vi "Platform.vi"() -> ()   [LabVIEW 2013]
uses:
  <vilib>/userdefined/High Color/IMAQdx.ctl
  <vilib>/Instr/_visa.llb/VISA Configure Serial Port (Instr).vi
  <vilib>/vision/driver/NI_Vision_Acquisition_Software.lvlib
  <vilib>/vision/NI_Vision_Development_Module.lvlib
panel:
  in  "VISA resource name 3":refnum<visa-resource-name>="COM13" caption="蓝牙串口选择"
  in  "baud rate  3":u16(ring)=9600 caption="蓝牙波特率设置" items=["115200"=0, "57600"=57600, "38400"=38400, "19200"=19200, "9600"=9600]
  out "x = y? 6":bool
  out "x = y? 5":bool
  out "x = y? 4":bool
  out "x = y? 3":bool
  out "x = y? 2":bool
  out "x = y?":bool
  out "数字":i32
  out "当前系统时间":string
  in  "系统总开关":bool
  out "x":i32 min=0 max=1 step=1
  out "检测目标总数目":dbl(knob) scale=0.0..10.0
  in  "连接确认":bool
  out "发送的坐标数据":string
  in  "过滤识别选项":u16(ring)=1 items=["过滤并分类摆放"=4, "过滤矩形目标"=3, "过滤圆形目标"=2, "全部识别"=1]
  in  "baud rate":u16(ring)=9600 caption="通讯波特率设置" items=["115200"=0, "57600"=57600, "38400"=38400, "19200"=19200, "9600"=9600]
  in  "VISA resource name":refnum<visa-resource-name>="COM3" caption="串口号选择"
  out "串口接收区：":string
  out "中间量":string
  in  "清空接收区":bool
  in  "关闭串口（调试）":bool
  in  "空载速率":dbl=1.0 min=1.0 max=3.0 step=1.0
  in  "运行速率":dbl=1.0 min=1.0 max=3.0 step=1.0
  in  "采集相机选择":T1="cam1"
  in  "环境光阈值设置":cluster{"环境光阈值设置":sgl, "上限值 value":sgl}={"环境光阈值设置"=137.0, "上限值 value"=255.0} {"环境光阈值设置" min=0 max=255 step=1 scale=0.0..255.0}
  out "图像处理后效果图":T2(plugin-control)
  out "捕捉画面":T2(plugin-control)
  in  "图像捕捉":bool
  out "监测画面":T2(plugin-control)
  # "基于机器视觉系统工业机器人控制平台   V5.0\n                             By Richard K    2014-03"
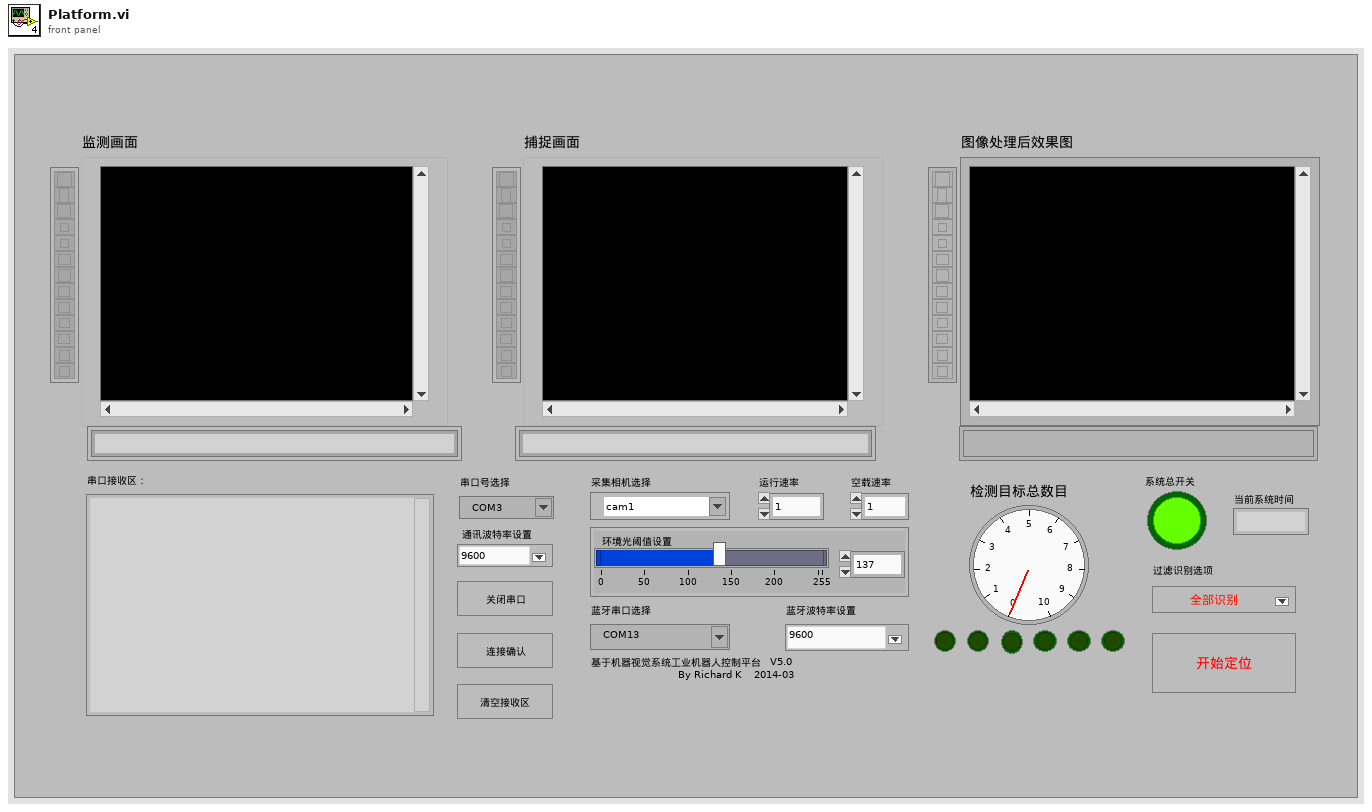
[diagram p1: front panel]
types:
  T1 = typedef "IMAQdx.ctl" = refnum<k21>
  T2 = typedef "IMAQ Image.ctl" = refnum<image>
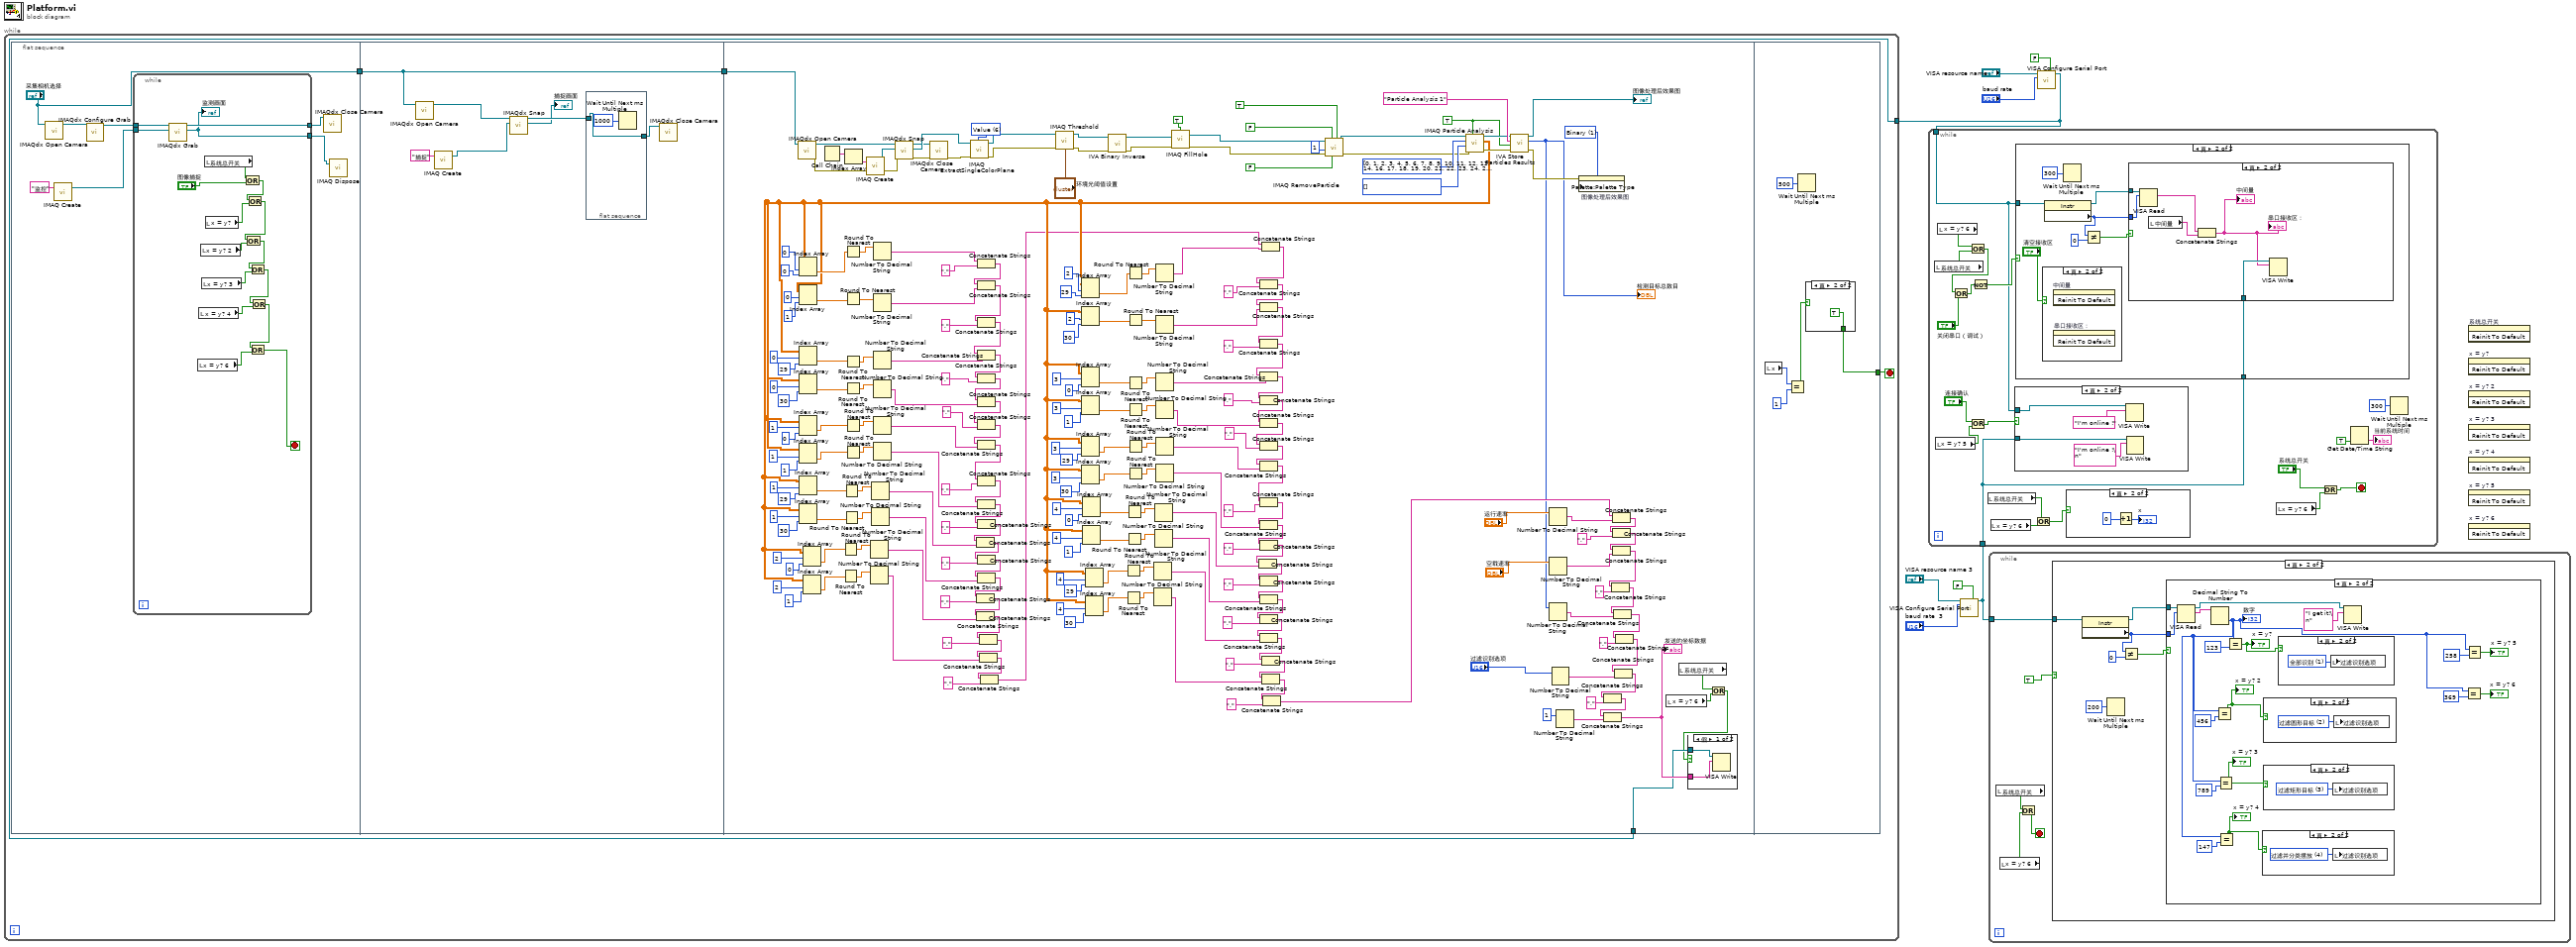
[diagram p0: block diagram]
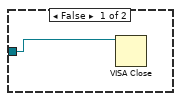
[diagram p2: hidden frame]
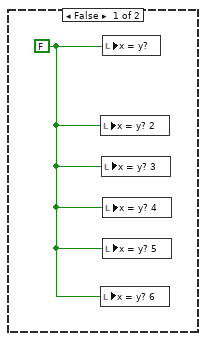
[diagram p3: hidden frame]
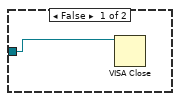
[diagram p10: hidden frame]
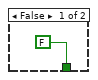
[diagram p14: hidden frame]
diagram:
  n1 = call-poly "VISA Configure Serial Port"("VISA resource name"="VISA resource name 3", "Enable Termination\nChar (T)"=FALSE ("Enable Termination\nChar (T)"), "baud rate (9600)"="baud rate  3") -> ("VISA resource name out"=w2:refnum<visa-resource-name>)  [unwired: 6 in, 6 out]
  n2 = while {
    tunnel: w2 -> [w13]
    stop <- w11 stop-if-true
    n3 = local read "系统总开关"() -> (w10:bool)
    n4 = local read "x = y? 6"() -> (w9:bool)
    n5 = Or(x=w10, y=w9) -> (x .or. y?=w11:bool)
    n6 = case shown="真" TRUE {
      tunnel: w13 -> [w14 w15]
      frame False {
        n7 = VISA Close(VISA resource name=w14) -> ()  [unwired: 1 in, 1 out]
      }
      frame True {
        n8 = property class="Instr"(reference=w15) -> (reference out=w17:refnum<visa-resource-name>, "Serial Settings:Number of Bytes at Serial Port"=w20:u32)  [unwired: 1 in, 1 out]
        n9 = Wait Until Next ms Multiple(millisecond multiple=u32 200 ("毫秒倍数")) -> ()  [unwired: 1 out]
        n10 = Not Equal?(x=w20, y=u32 0) -> (x != y?=w19:bool)
        n11 = case shown="真" w19 {
          tunnel: w17 -> [_ w39]
          tunnel: w20 -> [_ w38]
          frame False {
            w21 = FALSE ("x = y?")
            n12 = local write "x = y? 2"(w21) -> ()
            n13 = local write "x = y? 6"(w21) -> ()
            n14 = local write "x = y? 3"(w21) -> ()
            n15 = local write "x = y?"(w21) -> ()
            n16 = local write "x = y? 4"(w21) -> ()
            n17 = local write "x = y? 5"(w21) -> ()
          }
          frame True {
            n18 = VISA Read(VISA resource name=w39, byte count=w38) -> (VISA resource name out=w35:refnum<visa-resource-name>, read buffer=w37:string)  [unwired: 1 in, 2 out]
            n19 = Decimal String To Number(string=w37) -> (number=w22:i32)  [unwired: 2 in, 1 out]
            "数字" <- w22
            n20 = Equal?(x=w22, y=456) -> (x = y?=w28:bool)
            "x = y? 2" <- w28
            n21 = Equal?(x=w22, y=789) -> (x = y?=w29:bool)
            "x = y? 3" <- w29
            n22 = Equal?(x=w22, y=147) -> (x = y?=w27:bool)
            "x = y? 4" <- w27
            n23 = Equal?(x=w22, y=123) -> (x = y?=w33:bool)
            "x = y?" <- w33
            n24 = case shown="真" w27 {
              frame False {
              }
              frame True {
                w40 = u16 4 items=["过滤并分类摆放"=4, "过滤矩形目标"=3, "过滤圆形目标"=2, "全部识别"=1] ("过滤识别选项")
                n25 = local write "过滤识别选项"(w40) -> ()
              }
            }
            n26 = case shown="真" w28 {
              frame False {
              }
              frame True {
                w42 = u16 2 items=["过滤并分类摆放"=4, "过滤矩形目标"=3, "过滤圆形目标"=2, "全部识别"=1] ("过滤识别选项")
                n27 = local write "过滤识别选项"(w42) -> ()
              }
            }
            n28 = case shown="真" w29 {
              frame False {
              }
              frame True {
                w41 = u16 3 items=["过滤并分类摆放"=4, "过滤矩形目标"=3, "过滤圆形目标"=2, "全部识别"=1] ("过滤识别选项")
                n29 = local write "过滤识别选项"(w41) -> ()
              }
            }
            n30 = case shown="真" w33 {
              frame False {
              }
              frame True {
                w43 = u16 1 items=["过滤并分类摆放"=4, "过滤矩形目标"=3, "过滤圆形目标"=2, "全部识别"=1] ("过滤识别选项")
                n31 = local write "过滤识别选项"(w43) -> ()
              }
            }
            n32 = VISA Write(VISA resource name=w35, write buffer="I get it!\n" ("写入缓冲区")) -> ()  [unwired: 1 in, 3 out]
            n33 = Equal?(x=w22, y=369) -> (x = y?=→"x = y? 6":bool)
            n34 = Equal?(x=w22, y=258) -> (x = y?=→"x = y? 5":bool)
          }
        }
      }
    }
  }
  n35 = call-poly "VISA Configure Serial Port"("VISA resource name"="VISA resource name", "Enable Termination\nChar (T)"=FALSE ("Enable Termination\nChar (T)"), "baud rate (9600)"="baud rate") -> ("VISA resource name out"=w6:refnum<visa-resource-name>)  [unwired: 6 in, 6 out]
  n36 = while {
    tunnel: w6 -> [w45]
    stop <- w44 stop-if-true
    n37 = flat-sequence {
      tunnel: ["采集相机选择"] -> w47
      tunnel: w47 -> [w72]
      tunnel: [w72] -> w46
      tunnel: w46 -> [w268]
      tunnel: w45 -> [w84]
      tunnel: [w310] -> w44
      frame #0 {
        n38 = call <vilib>:"IMAQdx Open Camera.vi"("Session In"="采集相机选择") -> ("Session Out"=w54:T1)  [unwired: 9 in, 1 out]
        n39 = call "IMAQ Create"("Image Name"="监控") -> ("New Image"=w52:T2)  [unwired: 4 in, 1 out]
        n40 = call <vilib>:"IMAQdx Configure Grab.vi"("Session In"=w54) -> ("Session Out"=w51:T1)  [unwired: 9 in, 1 out]
        n41 = while {
          tunnel: w52 -> [w71]
          tunnel: w51 -> [w70]
          tunnel: [w69] -> w50
          tunnel: [w68] -> w49
          stop <- w55 stop-if-true
          n42 = call <vilib>:"IMAQdx Grab.vi"("Image In"=w71, "Session In"=w70) -> ("Image Out"=w68:T2, "Session Out"=w69:T1)  [unwired: 6 in, 2 out]
          "监测画面" <- w68
          n43 = local read "x = y? 6"() -> (w56:bool)
          n44 = local read "x = y? 4"() -> (w58:bool)
          n45 = local read "x = y? 2"() -> (w62:bool)
          n46 = local read "x = y? 3"() -> (w60:bool)
          n47 = local read "系统总开关"() -> (w67:bool)
          n48 = local read "x = y?"() -> (w64:bool)
          n49 = Or(x=w67, y="图像捕捉") -> (x .or. y?=w65:bool)
          n50 = Or(x=w65, y=w64) -> (x .or. y?=w63:bool)
          n51 = Or(x=w63, y=w62) -> (x .or. y?=w61:bool)
          n52 = Or(x=w61, y=w60) -> (x .or. y?=w59:bool)
          n53 = Or(x=w59, y=w58) -> (x .or. y?=w57:bool)
          n54 = Or(x=w57, y=w56) -> (x .or. y?=w55:bool)
        }
        n55 = call <vilib>:"IMAQdx Close Camera.vi"("Session In"=w50) -> ()  [unwired: 10 in, 1 out]
        n56 = call "IMAQ Dispose"("Image"=w49) -> ()  [unwired: 5 in, 1 out]
      }
      frame #1 {
        n57 = call <vilib>:"IMAQdx Open Camera.vi"("Session In"=w72) -> ("Session Out"=w77:T1)  [unwired: 9 in, 1 out]
        n58 = call "IMAQ Create"("Image Name"="捕捉") -> ("New Image"=w76:T2)  [unwired: 4 in, 1 out]
        n59 = call <vilib>:"IMAQdx Snap.vi"("Image In"=w76, "Session In"=w77) -> ("Image Out"=→"捕捉画面":T2, "Session Out"=w75:T1)  [unwired: 7 in, 1 out]
        n60 = flat-sequence {
          tunnel: [w79] -> w74
          tunnel: w75 -> [w79]
          frame #0 {
            n61 = Wait Until Next ms Multiple(millisecond multiple=u32 1000 ("毫秒倍数")) -> ()  [unwired: 1 out]
          }
        }
        n62 = call <vilib>:"IMAQdx Close Camera.vi"("Session In"=w74) -> ()  [unwired: 10 in, 1 out]
      }
      frame #2 {
        w304 = u32 1 items=["Grayscale", "Binary", "Gradient", "Rainbow", "Temperature", "User Defined"] ("Palette")
        w296 = i32[] [] items=["Center of Mass X", "Center of Mass Y", "First Pixel X", "First Pixel Y", "Bounding Rect Left", "Bounding Rect Top", "Bounding Rect Right", "Bounding Rect Bottom", "Max Feret Diameter Start X", "Max Feret Diameter Start Y", "Max Feret Diameter End X", "Max Feret Diameter End Y", "Max Horiz. Segment Length Left", "Max Horiz. Segment Length Right", "Max Horiz. Segment Length Row", "-", "Bounding Rect Width", "Bounding Rect Height", "Bounding Rect Diagonal", "Perimeter", "Convex Hull Perimeter", "Holes' Perimeter", "Max Feret Diameter", "Equivalent Ellipse Major Axis", "Equivalent Ellipse Minor Axis", "Equivalent Ellipse Minor Axis (Feret)", "Equivalent Rect Long Side", "Equivalent Rect Short Side", "Equivalent Rect Diagonal", "Equivalent Rect Short Side (Feret)", "Average Horiz. Segment Length", "Average Vert. Segment Length", "Hydraulic Radius", "Waddel Disk Diameter", "-", "Area", "Holes' Area", "Particle & Holes' Area", "Convex Hull Area", "Image Area", "-", "Number of Holes", "Number of Horiz. Segments", "Number of Vert. Segments", "-", "Orientation", "Max Feret Diameter Orientation", "-", "% Area/Image Area", "% Area/(Particle & Holes' Area)", "Ratio of Equivalent Ellipse Axes", "Ratio of Equivalent Rect Sides", "-", "Elongation Factor", "Compactness Factor", "Heywood Circularity Factor", "Type Factor", "-", "Sum X", "Sum Y", "Sum XX", "Sum XY", "Sum YY", "Sum XXX", "Sum XXY", "Sum XYY", "Sum YYY", "-", "Moment of Inertia XX", "Moment of Inertia XY", "Moment of Inertia YY", "Moment of Inertia XXX", "Moment of Inertia XXY", "Moment of Inertia XYY", "Moment of Inertia YYY", "Norm. Moment of Inertia XX", "Norm. Moment of Inertia XY", "Norm. Moment of Inertia YY", "Norm. Moment of Inertia XXX", "Norm. Moment of Inertia XXY", "Norm. Moment of Inertia XYY", "Norm. Moment of Inertia YYY", "Hu Moment 1", "Hu Moment 2", "Hu Moment 3", "Hu Moment 4", "Hu Moment 5", "Hu Moment 6", "Hu Moment 7"] ("Real-World Measurements")
        w295 = i32[] [0, 1, 2, 3, 4, 5, 6, 7, 8, 9, 10, 11, 12, 13, 14, 16, 17, 18, 19, 20, 21, 22, 23, 24, 25, 26, 27, 28, 29, 30, 31, 32, 33, 35, 36, 37, 38, 39, 41, 42, 43, 45, 46, 48, 49, 50, 51, 53, 54, 55, 56, 58, 59, 60, 61, 62, 63, 64, 65, 66, 68, 69, 70, 71, 72, 73, 74, 75, 76, 77, 78, 79, 80, 81, 82, 83, 84, 85, 86, 87, 88] items=["Center of Mass X", "Center of Mass Y", "First Pixel X", "First Pixel Y", "Bounding Rect Left", "Bounding Rect Top", "Bounding Rect Right", "Bounding Rect Bottom", "Max Feret Diameter Start X", "Max Feret Diameter Start Y", "Max Feret Diameter End X", "Max Feret Diameter End Y", "Max Horiz. Segment Length Left", "Max Horiz. Segment Length Right", "Max Horiz. Segment Length Row", "-", "Bounding Rect Width", "Bounding Rect Height", "Bounding Rect Diagonal", "Perimeter", "Convex Hull Perimeter", "Holes' Perimeter", "Max Feret Diameter", "Equivalent Ellipse Major Axis", "Equivalent Ellipse Minor Axis", "Equivalent Ellipse Minor Axis (Feret)", "Equivalent Rect Long Side", "Equivalent Rect Short Side", "Equivalent Rect Diagonal", "Equivalent Rect Short Side (Feret)", "Average Horiz. Segment Length", "Average Vert. Segment Length", "Hydraulic Radius", "Waddel Disk Diameter", "-", "Area", "Holes' Area", "Particle & Holes' Area", "Convex Hull Area", "Image Area", "-", "Number of Holes", "Number of Horiz. Segments", "Number of Vert. Segments", "-", "Orientation", "Max Feret Diameter Orientation", "-", "% Area/Image Area", "% Area/(Particle & Holes' Area)", "Ratio of Equivalent Ellipse Axes", "Ratio of Equivalent Rect Sides", "-", "Elongation Factor", "Compactness Factor", "Heywood Circularity Factor", "Type Factor", "-", "Sum X", "Sum Y", "Sum XX", "Sum XY", "Sum YY", "Sum XXX", "Sum XXY", "Sum XYY", "Sum YYY", "-", "Moment of Inertia XX", "Moment of Inertia XY", "Moment of Inertia YY", "Moment of Inertia XXX", "Moment of Inertia XXY", "Moment of Inertia XYY", "Moment of Inertia YYY", "Norm. Moment of Inertia XX", "Norm. Moment of Inertia XY", "Norm. Moment of Inertia YY", "Norm. Moment of Inertia XXX", "Norm. Moment of Inertia XXY", "Norm. Moment of Inertia XYY", "Norm. Moment of Inertia YYY", "Hu Moment 1", "Hu Moment 2", "Hu Moment 3", "Hu Moment 4", "Hu Moment 5", "Hu Moment 6", "Hu Moment 7"] ("Pixel Measurements")
        w298 = TRUE ("Connectivity 4/8 (8)")
        w279 = 6 items=["Red", "Green", "Blue", "Hue", "Saturation", "Luminance", "Value", "Intensity"] ("Color Plane")
        n63 = call <vilib>:"IMAQdx Open Camera.vi"("Session In"=w268) -> ("error out"=w270:errorcluster, "Session Out"=w276:T1)  [unwired: 2 in, 7 out]
        n64 = Call Chain() -> (call chain=w277:string[])
        n65 = Index Array(array=w277) -> (element=w278:string)  [unwired: 1 in]
        n66 = call "IMAQ Create"("Image Name"=w278, "error in (no error)"=w270) -> ("New Image"=w274:T2, "error out"=w275:errorcluster)  [unwired: 2 in, 1 out]
        n67 = call <vilib>:"IMAQdx Snap.vi"("error in"=w275, "Image In"=w274, "Session In"=w276) -> ("error out"=w272:errorcluster, "Image Out"=w280:T2, "Session Out"=w271:T1)  [unwired: 6 out]
        n68 = call <vilib>:"IMAQdx Close Camera.vi"("error in"=w272, "Session In"=w271) -> ("error out"=w273:errorcluster)  [unwired: 9 out]
        n69 = call "IMAQ ExtractSingleColorPlane"("Color Plane"=w279, "error in (no error)"=w273, "Image Src"=w280) -> ("error out"=w281:errorcluster, "Image Dst Out"=w282:T2)  [unwired: 1 in, 6 out]
        n70 = call "IMAQ Threshold"("error in (no error)"=w281, "Range"="环境光阈值设置", "Image Src"=w282) -> ("error out"=w283:errorcluster, "Image Dst Out"=w284:T2)  [unwired: 3 in, 4 out]
        n71 = call <vilib>:"IVA Binary Inverse.vi"("error in (no error)"=w283, "Image In"=w284) -> ("error out"=w285:errorcluster, "Image Out"=w287:T2)  [unwired: 8 out]
        n72 = call "IMAQ FillHole"("error in (no error)"=w285, "Image Src"=w287, "Connectivity 4/8 (8)"=TRUE) -> ("error out"=w288:errorcluster, "Image Dst Out"=w293:T2)  [unwired: 1 in, 2 out]
        n73 = call "IMAQ RemoveParticle"("Connectivity 4/8 (8)"=TRUE, "Low Pass/High Pass (Low)"=FALSE, "Square/Hexa (Square)"=FALSE, "error in (no error)"=w288, "Number of Erosion"=1, "Image Src"=w293) -> ("error out"=w294:errorcluster, "Image Dst Out"=w297:T2)  [unwired: 1 in, 3 out]
        n74 = call "IMAQ Particle Analysis"("Connectivity 4/8 (8)"=w298, "error in (no error)"=w294, "Real-World Measurements"=w296, "Pixel Measurements"=w295, "Image"=w297) -> ("error out"=w301:errorcluster, "Particle Measurements (Pixels)"=w101:dbl[][], "Image Out (duplicate)"=w299:T2)  [unwired: 4 out]
        n75 = Index Array(array=w101, index (row)=0 ("索引 (行)"), index (col)=0 ("禁用的索引 (列)")) -> (element=w260:dbl)
        n76 = Index Array(array=w101, index (row)=0 ("索引 (行)"), index (col)=1 ("禁用的索引 (列)")) -> (element=w256:dbl)
        n77 = Index Array(array=w101, index (row)=0 ("索引 (行)"), index (col)=29 ("禁用的索引 (列)")) -> (element=w238:dbl)
        n78 = Index Array(array=w101, index (row)=0 ("索引 (行)"), index (col)=30 ("禁用的索引 (列)")) -> (element=w237:dbl)
        n79 = Index Array(array=w101, index (row)=1 ("索引 (行)"), index (col)=0 ("禁用的索引 (列)")) -> (element=w236:dbl)
        n80 = Index Array(array=w101, index (row)=1 ("索引 (行)"), index (col)=1 ("禁用的索引 (列)")) -> (element=w235:dbl)
        n81 = Index Array(array=w101, index (row)=1 ("索引 (行)"), index (col)=29 ("禁用的索引 (列)")) -> (element=w200:dbl)
        n82 = Index Array(array=w101, index (row)=1 ("索引 (行)"), index (col)=30 ("禁用的索引 (列)")) -> (element=w199:dbl)
        n83 = Index Array(array=w101, index (row)=2 ("索引 (行)"), index (col)=0 ("禁用的索引 (列)")) -> (element=w198:dbl)
        n84 = Index Array(array=w101, index (row)=2 ("索引 (行)"), index (col)=1 ("禁用的索引 (列)")) -> (element=w197:dbl)
        n85 = Round To Nearest(number=w198) -> (nearest integer value=w202:dbl)
        n86 = Round To Nearest(number=w197) -> (nearest integer value=w201:dbl)
        n87 = Round To Nearest(number=w200) -> (nearest integer value=w203:dbl)
        n88 = Round To Nearest(number=w199) -> (nearest integer value=w204:dbl)
        n89 = Round To Nearest(number=w260) -> (nearest integer value=w259:dbl)
        n90 = Round To Nearest(number=w256) -> (nearest integer value=w255:dbl)
        n91 = Round To Nearest(number=w238) -> (nearest integer value=w234:dbl)
        n92 = Round To Nearest(number=w237) -> (nearest integer value=w233:dbl)
        n93 = Round To Nearest(number=w236) -> (nearest integer value=w232:dbl)
        n94 = Round To Nearest(number=w235) -> (nearest integer value=w231:dbl)
        n95 = Number To Decimal String(number=w202) -> (decimal integer string=w184:string)  [unwired: 1 in]
        n96 = Number To Decimal String(number=w201) -> (decimal integer string=w181:string)  [unwired: 1 in]
        n97 = Number To Decimal String(number=w203) -> (decimal integer string=w192:string)  [unwired: 1 in]
        n98 = Number To Decimal String(number=w204) -> (decimal integer string=w189:string)  [unwired: 1 in]
        n99 = Number To Decimal String(number=w259) -> (decimal integer string=w254:string)  [unwired: 1 in]
        n100 = Number To Decimal String(number=w255) -> (decimal integer string=w252:string)  [unwired: 1 in]
        n101 = Number To Decimal String(number=w234) -> (decimal integer string=w223:string)  [unwired: 1 in]
        n102 = Number To Decimal String(number=w233) -> (decimal integer string=w221:string)  [unwired: 1 in]
        n103 = Number To Decimal String(number=w232) -> (decimal integer string=w218:string)  [unwired: 1 in]
        n104 = Number To Decimal String(number=w231) -> (decimal integer string=w194:string)  [unwired: 1 in]
        n105 = Concatenate Strings(w254, ",") -> (w253:string)
        n106 = Concatenate Strings(w253, w252) -> (w266:string)
        n107 = Concatenate Strings(w266, ",") -> (w224:string)
        n108 = Concatenate Strings(w224, w223) -> (w222:string)
        n109 = Concatenate Strings(w222, ",") -> (w230:string)
        n110 = Concatenate Strings(w230, w221) -> (w227:string)
        n111 = Concatenate Strings(w227, ",") -> (w220:string)
        n112 = Concatenate Strings(w220, w218) -> (w219:string)
        n113 = Concatenate Strings(w219, ",") -> (w225:string)
        n114 = Concatenate Strings(w225, w194) -> (w193:string)
        n115 = Concatenate Strings(w193, ",") -> (w196:string)
        n116 = Concatenate Strings(w196, w192) -> (w191:string)
        n117 = Concatenate Strings(w191, ",") -> (w190:string)
        n118 = Concatenate Strings(w190, w189) -> (w186:string)
        n119 = Concatenate Strings(w186, ",") -> (w185:string)
        n120 = Concatenate Strings(w185, w184) -> (w183:string)
        n121 = Concatenate Strings(w183, ",") -> (w182:string)
        n122 = Concatenate Strings(w182, w181) -> (w179:string)
        n123 = Concatenate Strings(w179, ",") -> (w100:string)
        n124 = Index Array(array=w101, index (row)=2 ("索引 (行)"), index (col)=29 ("禁用的索引 (列)")) -> (element=w107:dbl)
        n125 = Index Array(array=w101, index (row)=2 ("索引 (行)"), index (col)=30 ("禁用的索引 (列)")) -> (element=w111:dbl)
        n126 = Index Array(array=w101, index (row)=3 ("索引 (行)"), index (col)=0 ("禁用的索引 (列)")) -> (element=w123:dbl)
        n127 = Index Array(array=w101, index (row)=3 ("索引 (行)"), index (col)=1 ("禁用的索引 (列)")) -> (element=w124:dbl)
        n128 = Index Array(array=w101, index (row)=3 ("索引 (行)"), index (col)=29 ("禁用的索引 (列)")) -> (element=w125:dbl)
        n129 = Index Array(array=w101, index (row)=3 ("索引 (行)"), index (col)=30 ("禁用的索引 (列)")) -> (element=w126:dbl)
        n130 = Index Array(array=w101, index (row)=4 ("索引 (行)"), index (col)=0 ("禁用的索引 (列)")) -> (element=w157:dbl)
        n131 = Index Array(array=w101, index (row)=4 ("索引 (行)"), index (col)=1 ("禁用的索引 (列)")) -> (element=w158:dbl)
        n132 = Index Array(array=w101, index (row)=4 ("索引 (行)"), index (col)=29 ("禁用的索引 (列)")) -> (element=w159:dbl)
        n133 = Index Array(array=w101, index (row)=4 ("索引 (行)"), index (col)=30 ("禁用的索引 (列)")) -> (element=w160:dbl)
        n134 = Round To Nearest(number=w159) -> (nearest integer value=w155:dbl)
        n135 = Round To Nearest(number=w160) -> (nearest integer value=w156:dbl)
        n136 = Round To Nearest(number=w157) -> (nearest integer value=w154:dbl)
        n137 = Round To Nearest(number=w158) -> (nearest integer value=w153:dbl)
        n138 = Round To Nearest(number=w107) -> (nearest integer value=w108:dbl)
        n139 = Round To Nearest(number=w111) -> (nearest integer value=w112:dbl)
        n140 = Round To Nearest(number=w123) -> (nearest integer value=w127:dbl)
        n141 = Round To Nearest(number=w124) -> (nearest integer value=w128:dbl)
        n142 = Round To Nearest(number=w125) -> (nearest integer value=w129:dbl)
        n143 = Round To Nearest(number=w126) -> (nearest integer value=w130:dbl)
        n144 = Number To Decimal String(number=w155) -> (decimal integer string=w173:string)  [unwired: 1 in]
        n145 = Number To Decimal String(number=w156) -> (decimal integer string=w176:string)  [unwired: 1 in]
        n146 = Number To Decimal String(number=w154) -> (decimal integer string=w165:string)  [unwired: 1 in]
        n147 = Number To Decimal String(number=w153) -> (decimal integer string=w168:string)  [unwired: 1 in]
        n148 = Number To Decimal String(number=w108) -> (decimal integer string=w99:string)  [unwired: 1 in]
        n149 = Number To Decimal String(number=w112) -> (decimal integer string=w114:string)  [unwired: 1 in]
        n150 = Number To Decimal String(number=w127) -> (decimal integer string=w138:string)  [unwired: 1 in]
        n151 = Number To Decimal String(number=w128) -> (decimal integer string=w140:string)  [unwired: 1 in]
        n152 = Number To Decimal String(number=w129) -> (decimal integer string=w143:string)  [unwired: 1 in]
        n153 = Number To Decimal String(number=w130) -> (decimal integer string=w163:string)  [unwired: 1 in]
        n154 = Concatenate Strings(w100, w99) -> (w98:string)
        n155 = Concatenate Strings(w98, ",") -> (w113:string)
        n156 = Concatenate Strings(w113, w114) -> (w102:string)
        n157 = Concatenate Strings(w102, ",") -> (w137:string)
        n158 = Concatenate Strings(w137, w138) -> (w139:string)
        n159 = Concatenate Strings(w139, ",") -> (w131:string)
        n160 = Concatenate Strings(w131, w140) -> (w134:string)
        n161 = Concatenate Strings(w134, ",") -> (w141:string)
        n162 = Concatenate Strings(w141, w143) -> (w142:string)
        n163 = Concatenate Strings(w142, ",") -> (w136:string)
        n164 = Concatenate Strings(w136, w163) -> (w164:string)
        n165 = Concatenate Strings(w164, ",") -> (w161:string)
        n166 = Concatenate Strings(w161, w165) -> (w166:string)
        n167 = Concatenate Strings(w166, ",") -> (w167:string)
        n168 = Concatenate Strings(w167, w168) -> (w171:string)
        n169 = Concatenate Strings(w171, ",") -> (w172:string)
        n170 = Concatenate Strings(w172, w173) -> (w174:string)
        n171 = Concatenate Strings(w174, ",") -> (w175:string)
        n172 = Concatenate Strings(w175, w176) -> (w178:string)
        n173 = Concatenate Strings(w178, ",") -> (w97:string)
        n174 = call <vilib>:"IVA Store Particles Results.vi"("error in (no error)"=w301, "Connectivity 4/8 (8)"=w298, "Step Name"="Particle Analysis 1", "Image in"=w299) -> ("error out"=w302:errorcluster, "Number of Particles"=w86:i32, "Image dup"=→"图像处理后效果图":T2)  [unwired: 5 out]
        "检测目标总数目" <- w86
        n175 = Number To Decimal String(number=w86) -> (decimal integer string=w213:string)  [unwired: 1 in]
        n176 = Number To Decimal String(number="运行速率") -> (decimal integer string=w267:string)  [unwired: 1 in]
        n177 = Number To Decimal String(number="空载速率") -> (decimal integer string=w247:string)  [unwired: 1 in]
        n178 = Number To Decimal String(number="过滤识别选项") -> (decimal integer string=w92:string)  [unwired: 1 in]
        n179 = Number To Decimal String(number=1 ("数字")) -> (decimal integer string=w89:string)  [unwired: 1 in]
        n180 = property on="图像处理后效果图" class="ImageControl"(error in=w302, "Palette:Palette Type"=w304) -> ()  [unwired: 1 in, 2 out]
        n181 = Concatenate Strings(w97, w267) -> (w250:string)
        n182 = Concatenate Strings(w250, ",") -> (w249:string)
        n183 = Concatenate Strings(w249, w247) -> (w215:string)
        n184 = Concatenate Strings(w215, ",") -> (w214:string)
        n185 = Concatenate Strings(w214, w213) -> (w94:string)
        n186 = Concatenate Strings(w94, ",") -> (w93:string)
        n187 = Concatenate Strings(w93, w92) -> (w88:string)
        n188 = Concatenate Strings(w88, ",") -> (w90:string)
        n189 = Concatenate Strings(w90, w89) -> (w85:string)
        "发送的坐标数据" <- w85
        n190 = local read "x = y? 6"() -> (w82:bool)
        n191 = local read "系统总开关"() -> (w83:bool)
        n192 = Or(x=w83, y=w82) -> (x .or. y?=w81:bool)
        n193 = case shown="假" w81 {
          tunnel: w85 -> [w306 _]
          tunnel: w84 -> [w305 _]
          frame False {
            n194 = VISA Write(VISA resource name=w305, write buffer=w306) -> ()  [unwired: 1 in, 3 out]
          }
          frame True {
          }
        }
      }
      frame #3 {
        n195 = local read "x"() -> (w307:i32)
        n196 = Equal?(x=w307, y=1) -> (x = y?=w309:bool)
        n197 = Wait Until Next ms Multiple(millisecond multiple=u32 500 ("毫秒倍数")) -> ()  [unwired: 1 out]
        n198 = case shown="真" w309 {
          tunnel: [FALSE TRUE] -> w310
          frame False {
          }
          frame True {
          }
        }
      }
    }
  }
  n199 = while {
    tunnel: w6 -> [w332]
    tunnel: w2 -> [w314]
    stop <- w321 stop-if-true
    n200 = local read "系统总开关"() -> (w316:bool)
    n201 = local read "x = y? 5"() -> (w324:bool)
    n202 = local read "x = y? 6"() -> (w317:bool)
    n203 = Or(x=w317, y=w316) -> (x .or. y?=w315:bool)
    n204 = Or(x=w315, y="关闭串口（调试）") -> (x .or. y?=w331:bool)
    n205 = Or(x="连接确认", y=w324) -> (x .or. y?=w325:bool)
    n206 = Not(x=w331) -> (.not. x?=w333:bool)
    n207 = local read "系统总开关"() -> (w318:bool)
    n208 = local read "x = y? 6"() -> (w320:bool)
    n209 = case shown="真" w325 {
      tunnel: w332 -> [_ w339]
      tunnel: w314 -> [_ w336]
      frame False {
      }
      frame True {
        n210 = VISA Write(VISA resource name=w339, write buffer="I'm online !" ("写入缓冲区")) -> ()  [unwired: 1 in, 3 out]
        n211 = VISA Write(VISA resource name=w336, write buffer="I'm online !\n" ("写入缓冲区")) -> ()  [unwired: 1 in, 3 out]
      }
    }
    n212 = case shown="真" w333 {
      tunnel: w332 -> [w340 w343]
      tunnel: w314 -> [_ w341]
      frame False {
        n213 = VISA Close(VISA resource name=w340) -> ()  [unwired: 1 in, 1 out]
      }
      frame True {
        n214 = case shown="真" "清空接收区" {
          frame False {
          }
          frame True {
            n215 = invoke on="中间量" class="Str" method="Reinit To Default"() -> ()  [unwired: 3 in, 3 out]
            n216 = invoke on="串口接收区：" class="Str" method="Reinit To Default"() -> ()  [unwired: 3 in, 3 out]
          }
        }
        n217 = property class="Instr"(reference=w343) -> (reference out=w345:refnum<visa-resource-name>, "Serial Settings:Number of Bytes at Serial Port"=w348:u32)  [unwired: 1 in, 1 out]
        n218 = Wait Until Next ms Multiple(millisecond multiple=u32 300 ("毫秒倍数")) -> ()  [unwired: 1 out]
        n219 = Not Equal?(x=w348, y=u32 0) -> (x != y?=w347:bool)
        n220 = case shown="真" w347 {
          tunnel: w345 -> [_ w354]
          tunnel: w348 -> [_ w353]
          tunnel: w341 -> [_ w350]
          frame False {
          }
          frame True {
            n221 = VISA Read(VISA resource name=w354, byte count=w353) -> (read buffer=w352:string)  [unwired: 1 in, 3 out]
            n222 = local read "中间量"() -> (w351:string)
            n223 = Concatenate Strings(w352, w351) -> (w349:string)
            "串口接收区：" <- w349
            "中间量" <- w349
            n224 = VISA Write(VISA resource name=w350, write buffer=w349) -> ()  [unwired: 1 in, 3 out]
          }
        }
      }
    }
    n225 = Or(x=w318, y=w320) -> (x .or. y?=w319:bool)
    n226 = case shown="真" w319 {
      frame False {
      }
      frame True {
        n227 = Increment(x=0) -> (x+1=→"x":i32)
      }
    }
    n228 = local read "x = y? 6"() -> (w323:bool)
    n229 = Or(x="系统总开关", y=w323) -> (x .or. y?=w321:bool)
    n230 = Get Date/Time String(want seconds? (F)=TRUE ("需要秒？(F)")) -> (time string=→"当前系统时间":string)  [unwired: 2 in, 1 out]
    n231 = Wait Until Next ms Multiple(millisecond multiple=u32 300 ("毫秒倍数")) -> ()  [unwired: 1 out]
  }
  n232 = invoke on="系统总开关" class="Bool (严格)" method="Reinit To Default"() -> ()  [unwired: 3 in, 3 out]
  n233 = invoke on="x = y?" class="Bool (严格)" method="Reinit To Default"() -> ()  [unwired: 3 in, 3 out]
  n234 = invoke on="x = y? 2" class="Bool (严格)" method="Reinit To Default"() -> ()  [unwired: 3 in, 3 out]
  n235 = invoke on="x = y? 3" class="Bool (严格)" method="Reinit To Default"() -> ()  [unwired: 3 in, 3 out]
  n236 = invoke on="x = y? 4" class="Bool (严格)" method="Reinit To Default"() -> ()  [unwired: 3 in, 3 out]
  n237 = invoke on="x = y? 5" class="Bool (严格)" method="Reinit To Default"() -> ()  [unwired: 3 in, 3 out]
  n238 = invoke on="x = y? 6" class="Bool (严格)" method="Reinit To Default"() -> ()  [unwired: 3 in, 3 out]
